vi "Indicator.vi"(4 "references of results":T2(array[cluster])) -> (0 "number of updates":i32[](array[numeric]), 1 "status":bool[](array[boolean]), 2 "results":T1[](array[typedef]))   [LabVIEW 2020]
uses:
  <userlib>/caLab/PV Info.ctl
  <userlib>/caLab/CaLab.lvlib
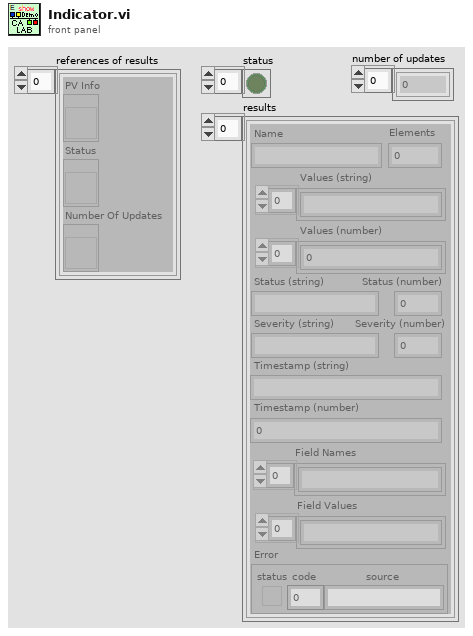
[diagram p1: front panel]
types:
  T1 = typedef "CaLab.lvlib/PV Info.ctl" = cluster{"Name":string, "Elements":i32, "Values (string)":string[], "Values (number)":dbl[], "Status (string)":string, "Status (number)":i16, "Severity (string)":string, "Severity (number)":i16, "Timestamp (string)":string, "Timestamp (number)":i32, "Field Names":string[], "Field Values":string[], "Error":errorcluster}
  T2 = cluster{"PV Info":refnum<vi>, "Status":refnum<vi>, "Number Of Updates":refnum<vi>}[]
  T3 = typedef "PV Info.ctl" = cluster{"Name":string, "Elements":i32, "Values (string)":string[], "Values (number)":dbl[], "Status (string)":string, "Status (number)":i16, "Severity (string)":string, "Severity (number)":i16, "Timestamp (string)":string, "Timestamp (number)":i32, "Field Names":string[], "Field Values":string[], "Error":errorcluster}
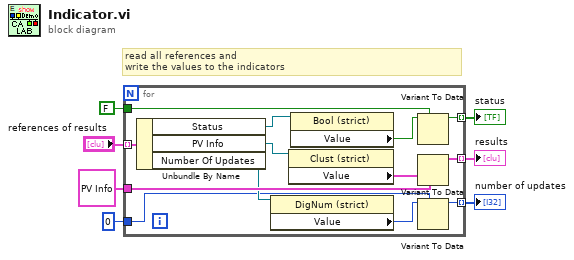
[diagram p0: block diagram]
diagram:
  # "read all references and\nwrite the values to the indicators"
  n1 = for {
    tunnel: [w18] -> w2 mode=indexing
    tunnel: [w17] -> w3 mode=indexing
    tunnel: [w12] -> w1 mode=indexing
    tunnel: T1 {"Name"="", "Elements"=0, "Values (string)"=[], "Values (number)"=[], "Status (string)"="", "Status (number)"=0, "Severity (string)"="", "Severity (number)"=0, "Timestamp (string)"="", "Timestamp (number)"=0, "Field Names"=[], "Field Values"=[], "Error"={"status"=FALSE, "code"=0, "source"=""}} ("PV Info x") -> [w16]
    tunnel: FALSE -> [w15]
    tunnel: 0 -> [w10]
    tunnel: "references of results" -> [w14] mode=indexing
    n2 = Unbundle By Name(w14) -> ("Status"=w9:refnum<vi>, "PV Info"=w8:refnum<vi>, "Number Of Updates"=w13:refnum<vi>)
    n3 = property class="DigNum (strict)"(reference=w13) -> ("Value"=w11:i32)  [unwired: 1 in, 2 out]
    n4 = property class="Clust (strict)"(reference=w8) -> ("Value"=w19:T3)  [unwired: 1 in, 2 out]
    n5 = property class="Bool (strict)"(reference=w9) -> ("Value"=w20:bool)  [unwired: 1 in, 2 out]
    n6 = Variant To Data(type=w15, Variant=w20) -> (data=w17:bool)  [unwired: 1 in, 1 out]
    n7 = Variant To Data(type=w16, Variant=w19) -> (data=w18:T1)  [unwired: 1 in, 1 out]
    n8 = Variant To Data(type=w10, Variant=w11) -> (data=w12:i32)  [unwired: 1 in, 1 out]
  }
  "status" <- w3
  "results" <- w2
  "number of updates" <- w1
